vi "main2.vi"() -> ()   [LabVIEW 2019]
panel:
  out "y ideal chegada":dbl
  out "x ideal chegada":dbl
  out "y ideal partida":dbl
  out "x ideal partida":dbl
  out "y real chegada":dbl
  out "x real chegada":dbl
  out "y real partida":dbl
  out "x real partida":dbl
  out "erro percentual do x final":dbl
  out "erro percentual do x inicial":dbl
  out "erro percentual do y inicial":dbl
  out "erro percentual do y final":dbl
  in  "ideal":path=path "adp.csv"
  in  "real":path=path "adp.csv"
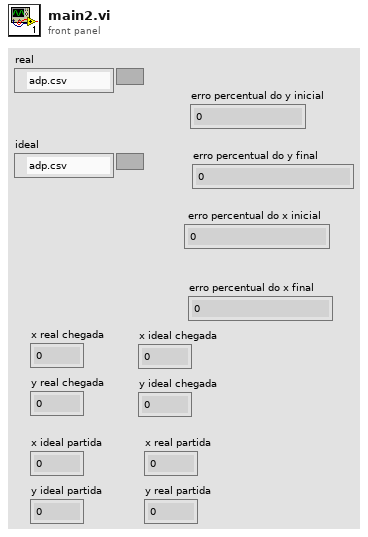
[diagram p1: front panel]
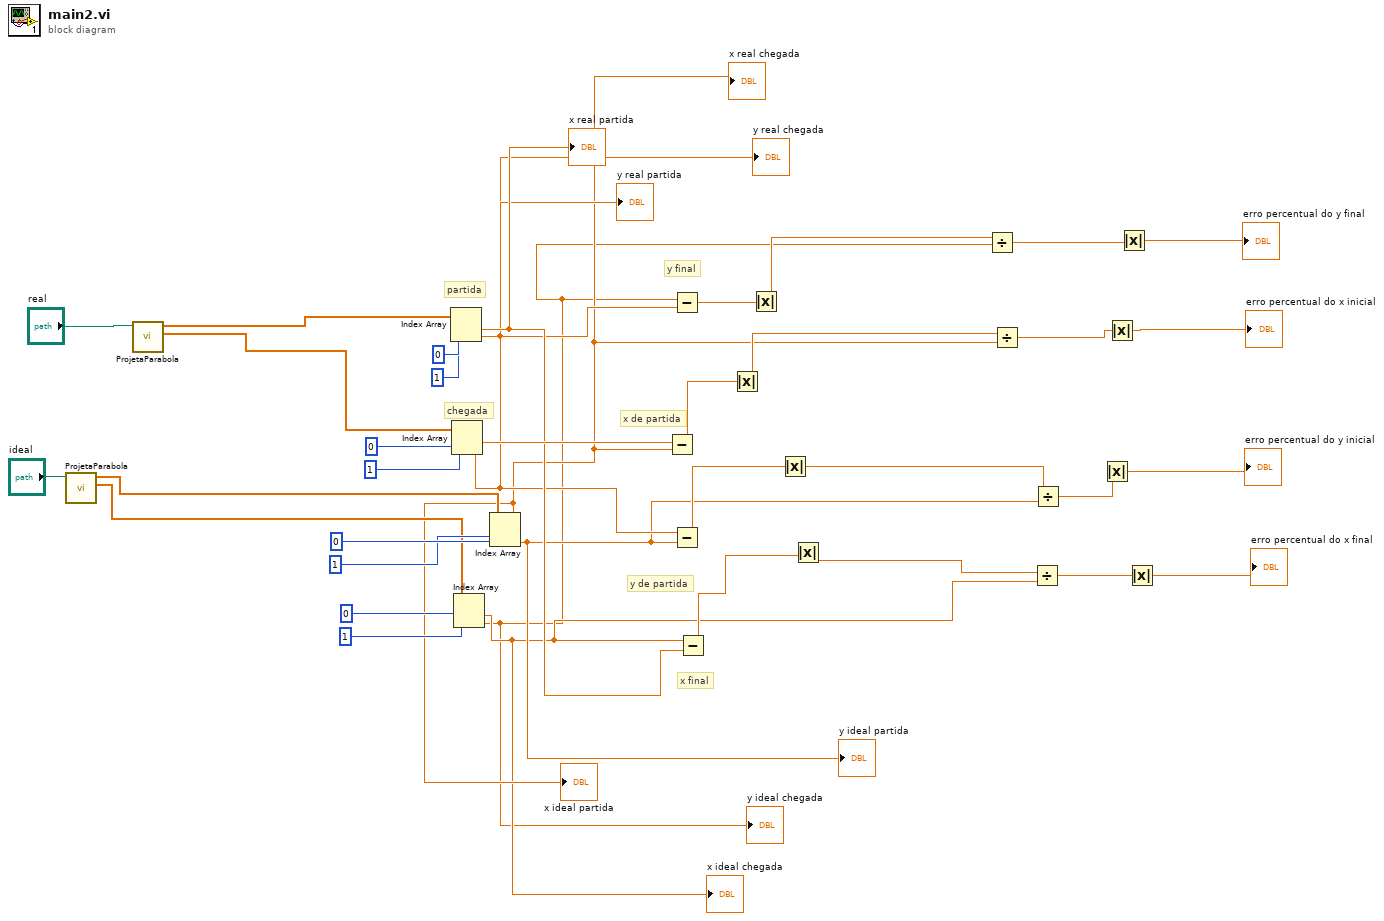
[diagram p0: block diagram]
diagram:
  # "chegada"
  # "partida"
  # "y final"
  # "x final"
  # "y de partida"
  # "x de partida"
  n1 = call "ProjetaParabola.vi"("file path (dialog if empty)"="ideal") -> ("chegada"=w6:dbl[], "partida"=w7:dbl[])  [unwired: 9 in]
  n2 = call "ProjetaParabola.vi"("file path (dialog if empty)"="real") -> ("chegada"=w9:dbl[], "partida"=w10:dbl[])  [unwired: 9 in]
  n3 = Index Array(array=w10, index #1=0, index #2=1) -> (element #1=w22:dbl, element #2=w21:dbl)
  "x real partida" <- w22
  "y real partida" <- w21
  n4 = Index Array(array=w9, index #1=0, index #2=1) -> (element #1=w29:dbl, element #2=w5:dbl)
  "y real chegada" <- w5
  n5 = Index Array(array=w6, index #1=0, index #2=1) -> (element #1=w2:dbl, element #2=w1:dbl)
  "x ideal chegada" <- w2
  "y ideal chegada" <- w1
  n6 = Index Array(array=w7, index #1=0, index #2=1) -> (element #1=w4:dbl, element #2=w3:dbl)
  "x real chegada" <- w4
  "x ideal partida" <- w4
  "y ideal partida" <- w3
  n7 = Subtract(x=w29, y=w4) -> (x-y=w27:dbl)
  n8 = Subtract(x=w1, y=w21) -> (x-y=w28:dbl)
  n9 = Subtract(x=w5, y=w3) -> (x-y=w26:dbl)
  n10 = Subtract(x=w2, y=w22) -> (x-y=w24:dbl)
  n11 = Absolute Value(x=w27) -> (abs(x)=w23:dbl)
  n12 = Absolute Value(x=w28) -> (abs(x)=w25:dbl)
  n13 = Absolute Value(x=w26) -> (abs(x)=w11:dbl)
  n14 = Absolute Value(x=w24) -> (abs(x)=w12:dbl)
  n15 = Divide(x=w25, y=w1) -> (x/y=w14:dbl)
  n16 = Divide(x=w23, y=w4) -> (x/y=w16:dbl)
  n17 = Divide(x=w12, y=w2) -> (x/y=w20:dbl)
  n18 = Divide(x=w11, y=w3) -> (x/y=w18:dbl)
  n19 = Absolute Value(x=w18) -> (abs(x)=→"erro percentual do y inicial":dbl)
  n20 = Absolute Value(x=w16) -> (abs(x)=→"erro percentual do x inicial":dbl)
  n21 = Absolute Value(x=w14) -> (abs(x)=→"erro percentual do y final":dbl)
  n22 = Absolute Value(x=w20) -> (abs(x)=→"erro percentual do x final":dbl)
